vi "ep_Check Size and Positions.vi"(8 "error in (no error)":errorcluster, 11 "resampled data":T1[](array[typedef]) {"resampled signal" format="%.2f"; "positions [s]" format="%.2f"}) -> (0 "error out":errorcluster, 1 "resampled signal":dbl[][](array[numeric]), 3 "positions [s]":dbl[](array[numeric]))   [LabVIEW 2013, in "NI_EP_Power Measurement.lvlib"]
uses:
  <vilib>/addons/Electrical Power/Power Measurement/NI_EP_Power Measurement.lvlib
  <vilib>/addons/Electrical Power/Power Measurement/subVIs/ep_Resampled Data.ctl
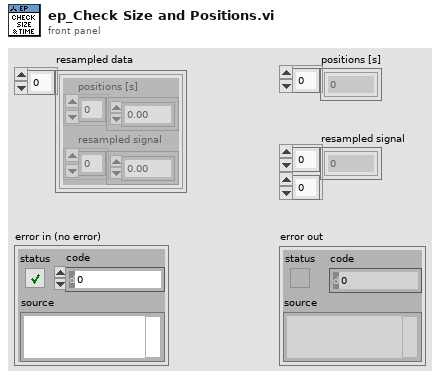
[diagram p1: front panel]
types:
  T1 = typedef "NI_EP_Power Measurement.lvlib/ep_Resampled Data.ctl" = cluster{"positions [s]":dbl[], "resampled signal":dbl[]}
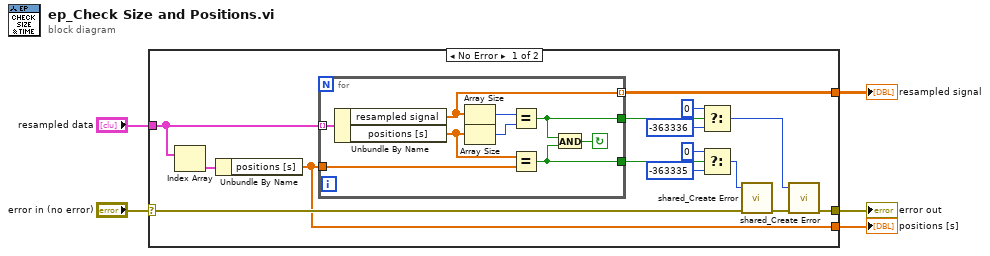
[diagram p0: block diagram]
diagram:
  n1 = case shown="No Error" "error in (no error)" {
    selector: "error in (no error)" -> [w17 w30]
    tunnel: [w9 w30] -> w4
    tunnel: "resampled data" -> [w16 _]
    tunnel: [w7 _] -> w2
    tunnel: [w6 _] -> w1
    frame No Error {
      n2 = Index Array(array=w16) -> (element=w15:T1)  [unwired: 1 in]
      n3 = Unbundle By Name(w15) -> ("positions [s]"=w6:dbl[])
      n4 = for {
        tunnel: w16 -> [w29] mode=indexing
        tunnel: w6 -> [w25]
        tunnel: [w23] -> w11
        tunnel: [w21] -> w14
        tunnel: [w22] -> w7 mode=indexing
        stop <- w24 continue-if-true
        n5 = Unbundle By Name(w29) -> ("resampled signal"=w22:dbl[], "positions [s]"=w26:dbl[])
        n6 = Array Size(array=w22) -> (size(s)=w28:i32)
        n7 = Array Size(array=w26) -> (size(s)=w27:i32)
        n8 = Equal?(x=w28, y=w27) -> (x = y?=w23:bool)
        n9 = Equal?(x=w26, y=w25) -> (x = y?=w21:bool)
        n10 = And(x=w23, y=w21) -> (x .and. y?=w24:bool)
      }
      n11 = Select(t=0 ("error code (0)"), s=w11, f=-363336 ("error code (0)")) -> (s? t:f=w8:i32)
      n12 = Select(t=0 ("error code (0)"), s=w14, f=-363335 ("error code (0)")) -> (s? t:f=w18:i32)
      n13 = call <vilib>:"shared_Create Error.vi"("error in (no error)"=w17, "error code (0)"=w18) -> ("error out"=w10:errorcluster)  [unwired: 9 in]
      n14 = call <vilib>:"shared_Create Error.vi"("error in (no error)"=w10, "error code (0)"=w8) -> ("error out"=w9:errorcluster)  [unwired: 9 in]
    }
    frame Error {
    }
  }
  "error out" <- w4
  "positions [s]" <- w1
  "resampled signal" <- w2
